vi "_meas_Ic2_by_volt.vi"(6 "Bias_LO_equip":T1={"Node address"=19, "CAN Interface"="CAN0", "Cartridge band"=10, "Slave Node in"={"Address"=19, "Serial Number"=[16, 71, 55, 76, 1, 8, 0, -15]}, "ObjHandle out"=89653312, "POL"=1, "sb"=1, "GPIB_SM (SIS S,V)"="24", "GPIB_DMM (SIS I)"="22", "GPIB_SM (MAG I) "="25", "GPIB_SG(LO)"="19", "GPIB_PW (PAMP) "="6", "GPIB_TMP1(8ch)"="12", "GPIB_TMP2(2ch)  "="13", "WCA_avg"=10, "Rsen"=10.0, "BiasModule"=0, "LOModule "=1, "WCA_LO_FREQ_SET"={"YTO Low freq. [GHz]"=14.42, "YTO High freq. [GHz]"=17.7, "Kvco"=1, "Lock Pol."=0, "SET LO FREQ"=72.5, "Multiplier"=6.0, "YTO (HEX)"=0, "YTO coarse( FREQ)"=25.0, "NULL PLL INTEGRATOR"=FALSE}, "Res for"=0} {"Res for" items=["none", "series res", "parallel res"]; "WCA_LO_FREQ_SET"."YTO coarse( FREQ)" min=25 max=150 step=0.0001 format="%.3f"; "WCA_LO_FREQ_SET"."Multiplier" min=3 max=6 step=3; "WCA_LO_FREQ_SET"."SET LO FREQ" min=25 max=150 step=0.0001 format="%.3f"; "WCA_LO_FREQ_SET"."Lock Pol." items=["Lower", "Upper"]; "WCA_LO_FREQ_SET"."Kvco" items=["7.5MHz/V", "15MHz/V"]; "WCA_LO_FREQ_SET"."YTO High freq. [GHz]" format="%.3f"; "WCA_LO_FREQ_SET"."YTO Low freq. [GHz]" format="%.3f"; "LOModule" items=["Manual", "B10Lab LO", "WCA LO"]; "BiasModule" items=["B10Lab Bias", "WCA BiasModule"]; "Slave Node in"."Serial Number" format="%.0x"; "Slave Node in"."Address" format="%.0x"; "Cartridge band" max=10 step=1; "Node address" format="%.0x"}, 7 "Icクラスタ":cluster{"start":dbl, "stop":dbl, "step":dbl}={"start"=-0.1, "stop"=2.5, "step"=0.05}) -> (3 "IC":dbl=2.000000000000001)   [LabVIEW 2017]
uses:
  <vilib>/express/express arith-compare/Formula/XNode/ExpressFormulaBlockNode.xnode
panel:
  out "XYグラフ":cluster{dbl[], dbl[]}(graph)
  # "LO freq. [GHz]"
  # "YTO LOW\n/High Freq."
  # "ZERO Intgrtr"
  # "Node Address"
  # "Serial Number"
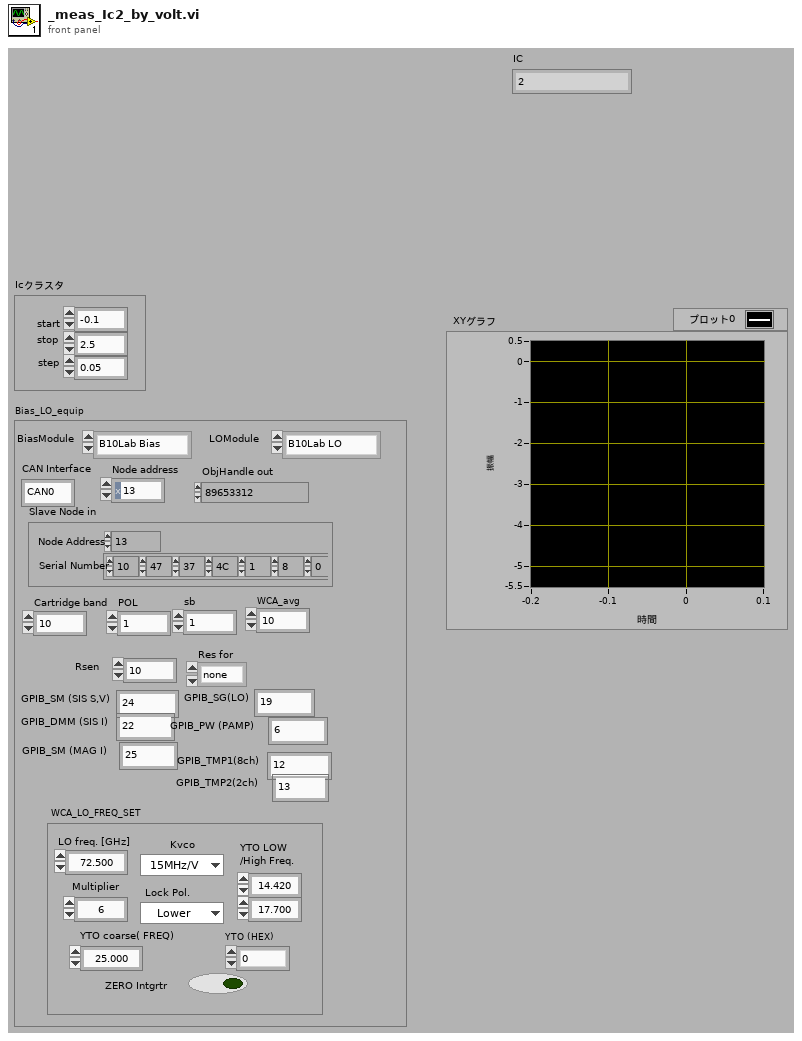
[diagram p1: front panel]
types:
  T1 = cluster{"Node address":u16, "CAN Interface":string, "Cartridge band":u32, "Slave Node in":cluster{"Address":i16, "Serial Number":i8[]}, "ObjHandle out":u32, "POL":u32, "sb":u32, "GPIB_SM (SIS S,V)":string, "GPIB_DMM (SIS I)":string, "GPIB_SM (MAG I) ":string, "GPIB_SG(LO)":string, "GPIB_PW (PAMP) ":string, "GPIB_TMP1(8ch)":string, "GPIB_TMP2(2ch)  ":string, "WCA_avg":i32, "Rsen":dbl, "BiasModule":u16, "LOModule ":u16, "WCA_LO_FREQ_SET":cluster{"YTO Low freq. [GHz]":sgl, "YTO High freq. [GHz]":sgl, "Kvco":u16, "Lock Pol.":u16, "SET LO FREQ":sgl, "Multiplier":sgl, "YTO (HEX)":u16, "YTO coarse( FREQ)":sgl, "NULL PLL INTEGRATOR":bool}, "Res for":u16}
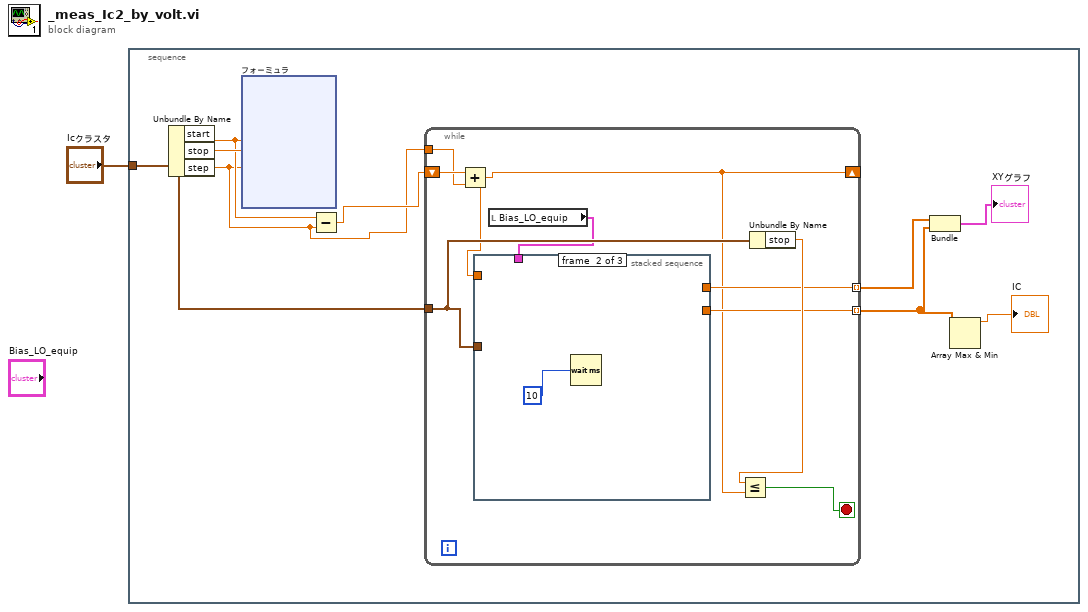
[diagram p0: block diagram]
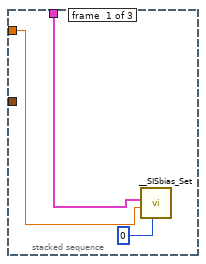
[diagram p2: hidden frame]
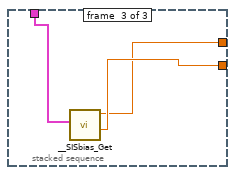
[diagram p3: hidden frame]
diagram:
  n1 = stacked-sequence {
    tunnel: "Icクラスタ" -> [w9]
    frame #0 {
      n2 = Unbundle By Name(w9) -> ("start"=w8:dbl, "stop"=w10:dbl, "step"=w6:dbl)
      n3 = xnode "フォーミュラ"("start"=w8, "stop"=w10, "step"=w6) -> ()  [unwired: 1 in, 2 out]
      n4 = Subtract(x=w8, y=w6) -> (x-y=w7:dbl)
      n5 = while {
        shift-right: [w24] -> _
        shift-left: w7 -> [w31]
        tunnel: w6 -> [w30]
        tunnel: w9 -> [w29]
        tunnel: [w26] -> w3 mode=indexing
        tunnel: [w25] -> w4 mode=indexing
        stop <- w23 stop-if-true
        n6 = Add(x=w31, y=w30) -> (x+y=w24:dbl)
        n7 = local read "Bias_LO_equip"() -> (w27:T1)
        n8 = stacked-sequence {
          tunnel: w24 -> [w34 _ _]
          tunnel: [_ _ w37] -> w26
          tunnel: w29 -> [_ _ _]
          tunnel: w27 -> [w32 _ w38]
          tunnel: [_ _ w36] -> w25
          frame #0 {
            n9 = call "__SISbias_Set.vi"("SIS　Mode"=0, "Set_V"=w34, "Bias_LO_equip"=w32) -> ()  [unwired: 8 in, 1 out]
          }
          frame #1 {
            n10 = Wait (ms)(milliseconds to wait=10) -> ()  [unwired: 1 out]
          }
          frame #2 {
            n11 = call "__SISbias_Get.vi"("Bias_LO_equip"=w38) -> ("Get_I(uA)"=w37:dbl, "Get_V(mV)"=w36:dbl)  [unwired: 8 in, 1 out]
          }
        }
        n12 = Unbundle By Name(w29) -> ("stop"=w28:dbl)
        n13 = Less Or Equal?(x=w28, y=w24) -> (x <= y?=w23:bool)
      }
      n14 = Bundle(w4, w3) -> (→"XYグラフ":cluster{dbl[], dbl[]})  [unwired: 1 in]
      n15 = Array Max & Min(array=w3) -> (max value=→"IC":dbl)  [unwired: 3 out]
    }
  }
